vi "GUILib.simple numeric init.vi"(0 "ctlRef":refnum<vi>, 2 "increment":dbl=1.0, 5 "error in (no error)":errorcluster) -> (14 "ctlRef dup":refnum<vi>, 19 "error out":errorcluster)   [LabVIEW 2012, in "GUILib.lvlib"]
doc: "initialiazes a specific type of control by setting default values"
uses:
  GUILib.lvlib
  UtilityLib/UtilityLib.valueStatus.ctl
  UtilityLib/UtilityLib.lvlib
panel:
  in  "numericType":dbl step=22.0
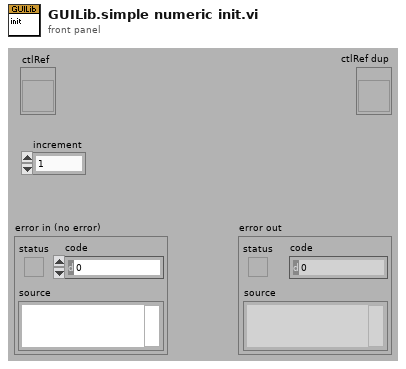
[diagram p1: front panel]
types:
  T1 = typedef "UtilityLib.lvlib/UtilityLib.valueStatus.ctl" = enum16{"no info available", "stand by/off", "on", "warning", "alarm/malfunction", "not implemented", "user action required", "important information", "system default", "control default", "indicator default", "button default"}
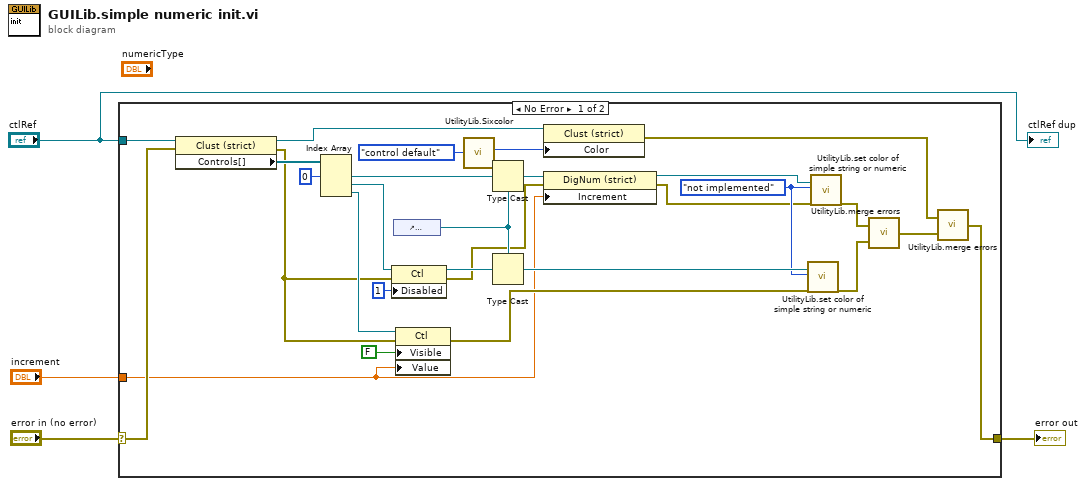
[diagram p0: block diagram]
diagram:
  n1 = case shown="No Error" "error in (no error)" {
    selector: "error in (no error)" -> [w19 w33]
    tunnel: "ctlRef" -> [w24 _]
    tunnel: "increment" -> [w9 _]
    tunnel: [w5 w33] -> w2
    frame No Error {
      w23 = UtilityLib.valueStatus."not implemented" ("valueStatus")
      n2 = property on="Property Node" class="Clust (strict)"(reference=w24, error in=w19) -> (reference out=w12:refnum<vi>, error out=w18:errorcluster, "Controls[]"=w25:refnum<vi>[])
      n3 = Index Array(array=w25, index #1=0 ("index")) -> (element #1=w29:refnum<vi>, element #2=w31:refnum<vi>, element #3=w22:refnum<vi>)  [unwired: 2 in]
      n4 = property class="Ctl"(reference=w31, error in=w18, "Disabled"=u8 1) -> (reference out=w32:refnum<vi>, error out=w17:errorcluster)
      n5 = control-ref of="numericType"() -> (w30:refnum<vi>)
      n6 = property class="Ctl"(reference=w22, error in=w18, "Visible"=FALSE, "Value"=w9) -> (error out=w15:errorcluster)  [unwired: 1 out]
      n7 = call "UtilityLib.Sixcolor.vi"("State"=UtilityLib.valueStatus."control default") -> ("elementBackground"=w11:u32)  [unwired: 2 in, 3 out]
      n8 = Type Cast(type=w30, x=w29) -> (*(type *) &x=w21:refnum<vi>)
      n9 = Type Cast(type=w30, x=w32) -> (*(type *) &x=w28:refnum<vi>)
      n10 = property on="Property Node" class="Clust (strict)"(reference=w12, "Color"=w11) -> (error out=w7:errorcluster)  [unwired: 1 in, 1 out]
      n11 = property class="DigNum (strict)"(reference=w21, error in=w17, "Increment"=w9) -> (reference out=w20:refnum<vi>, error out=w16:errorcluster)
      n12 = call "UtilityLib.set color of simple string or numeric.vi"("simpleNumeric"=w28, "valueStatus"=w23, "error in (no error)"=w15) -> ("error out"=w13:errorcluster)  [unwired: 16 in]
      n13 = call "UtilityLib.set color of simple string or numeric.vi"("simpleNumeric"=w20, "valueStatus"=w23, "error in (no error)"=w16) -> ("error out"=w14:errorcluster)  [unwired: 16 in]
      n14 = call "UtilityLib.merge errors.vi"("error2 (no error)"=w13, "error1 (no error)"=w14) -> ("error out"=w6:errorcluster)
      n15 = call "UtilityLib.merge errors.vi"("error2 (no error)"=w6, "error1 (no error)"=w7) -> ("error out"=w5:errorcluster)
    }
    frame Error {
    }
  }
  "error out" <- w2
  "ctlRef dup" <- "ctlRef"
